vi "cosinussinus.vi"() -> ()   [LabVIEW 2015]
panel:
  in  "stop":bool
  out "Waveform Chart":dbl[](graph)
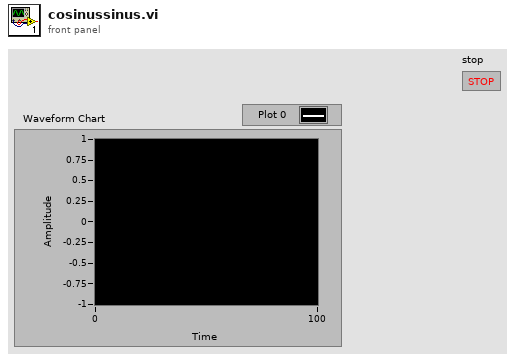
[diagram p1: front panel]
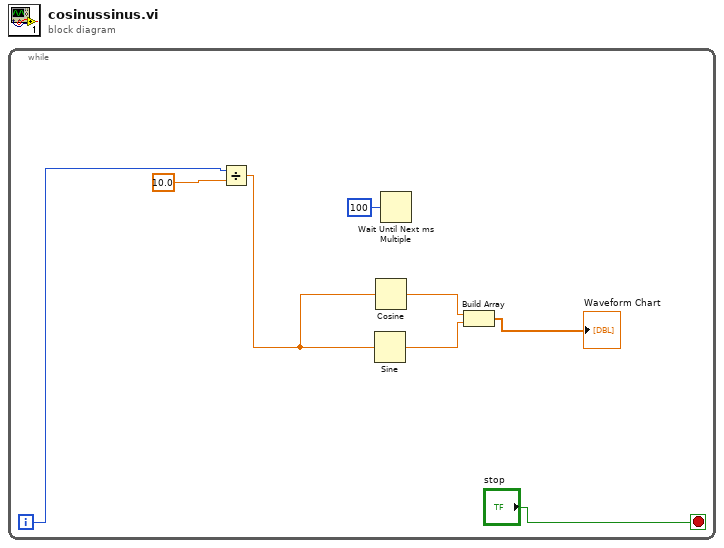
[diagram p0: block diagram]
diagram:
  n1 = while {
    i -> [w7]
    stop <- "stop" stop-if-true
    n2 = Divide(x=w7, y=10.0) -> (x/y=w6:dbl)
    n3 = Sine(x=w6) -> (sin(x)=w4:dbl)
    n4 = Cosine(x=w6) -> (cos(x)=w5:dbl)
    n5 = Wait Until Next ms Multiple(millisecond multiple=u32 100) -> ()  [unwired: 1 out]
    n6 = Build Array(w5, w4) -> (→"Waveform Chart":dbl[])
  }
